vi "remove353.vi"(8 "error in (no error)":errorcluster, 11 "Value in":refnum<class "Value.lvclass">) -> (0 "error out":errorcluster, 3 "Value out":refnum<class "Value.lvclass">)   [LabVIEW 2023]
uses:
  Value.lvclass
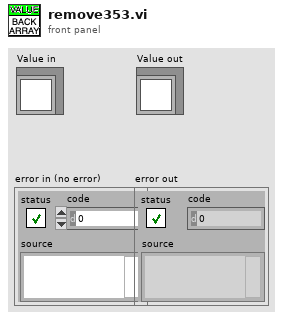
[diagram p1: front panel]
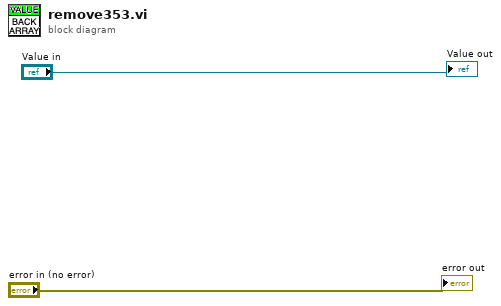
[diagram p0: block diagram]
diagram:
  "error out" <- "error in (no error)"
  "Value out" <- "Value in"
